vi "Change Font Colour.vi"(11 "valid?":bool) -> (3 "font colour":u32)   [LabVIEW 2021, in "MeasurementClient Editor.lvlib"]
uses:
  MeasurementClient Editor.lvlib
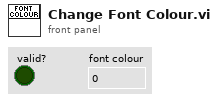
[diagram p1: front panel]
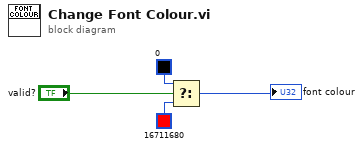
[diagram p0: block diagram]
diagram:
  n1 = Select(t=u32 0 ("Active Cell:Cell Font:Color"), s="valid?", f=u32 16711680 ("Active Cell:Cell Font:Color")) -> (s? t:f=→"font colour":u32)
